vi "PRIME Detector Process Images.vi"(8 "error in (no error)":errorcluster, 11 "prime detector status":T1) -> (0 "error out":errorcluster, 3 "Images":T2[](array[typedef]) {"Detector #" items=["None", "YJ", "HK"]})   [LabVIEW 2021, in "PRIME Detector.lvclass"]
uses:
  PRIME Detector.lvclass
  Detector Image typedef cluster.ctl
  PRIME Detector cluster Status.ctl
  Detector Class.lvclass
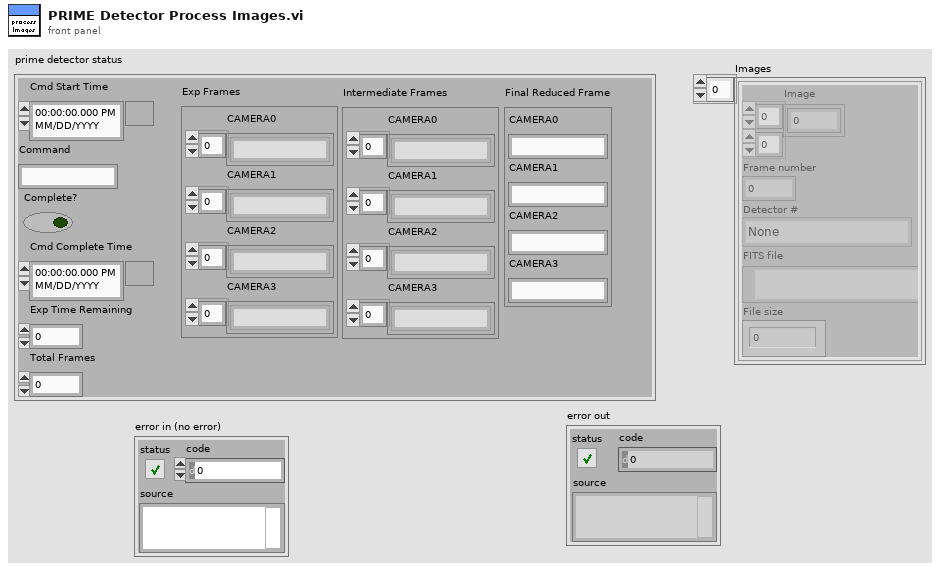
[diagram p1: front panel]
types:
  T1 = typedef "PRIME Detector cluster Status.ctl" = cluster{"Cmd Start Time":timestamp, "Command":string, "Complete?":bool, "Cmd Complete Time":timestamp, "Exp Time Remaining":dbl, "Total Frames":i32, "Exp Frames":cluster{"CAMERA0":string[], "CAMERA1":string[], "CAMERA2":string[], "CAMERA3":string[]}, "Intermediate Frames":cluster{"CAMERA0":string[], "CAMERA1":string[], "CAMERA2":string[], "CAMERA3":string[]}, "Final Reduced Frame":cluster{"CAMERA0":string, "CAMERA1":string, "CAMERA2":string, "CAMERA3":string}}
  T2 = typedef "Detector Class.lvclass/Detector Image typedef cluster.ctl" = cluster{"Image":sgl[][], "Frame number":i32, "Detector #":u16, "FITS file":path, "File size":i64}
  T3 = cluster{"CAMERA0":string[], "CAMERA1":string[], "CAMERA2":string[], "CAMERA3":string[]}
  T4 = cluster{"CAMERA0":string, "CAMERA1":string, "CAMERA2":string, "CAMERA3":string}
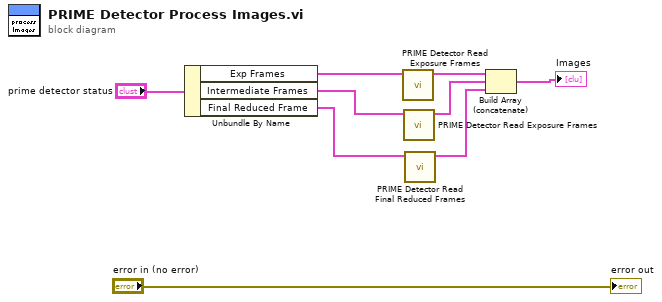
[diagram p0: block diagram]
diagram:
  n1 = Unbundle By Name("prime detector status") -> ("Exp Frames"=w9:T3, "Intermediate Frames"=w8:T3, "Final Reduced Frame"=w7:T4)
  n2 = call "PRIME Detector Read Exposure Frames.vi"("Exp Frames"=w9) -> ("Images"=w6:T2[])  [unwired: 10 in]
  n3 = call "PRIME Detector Read Exposure Frames.vi"("Exp Frames"=w8) -> ("Images"=w5:T2[])  [unwired: 10 in]
  n4 = call "PRIME Detector Read Final Reduced Frames.vi"("Final Reduced Frame"=w7) -> ("Images"=w4:T2[])  [unwired: 10 in]
  n5 = Build Array (concatenate)(w6, w5, w4) -> (→"Images":T2[])
  "error out" <- "error in (no error)"
